vi "feedback.vi"(3 "Dataflow In":errorcluster) -> (1 "Dataflow Out":errorcluster)   [LabVIEW 2019]
uses:
  lib/libSimulationControl/libSimulationControl.lvlib
panel:
  # "*******************************************************************\nBiogas Plant Control\n\nAuthor: Paul Zügel\nGCSC-Frankfurt am Main 2020\n\n*******************************************************************"
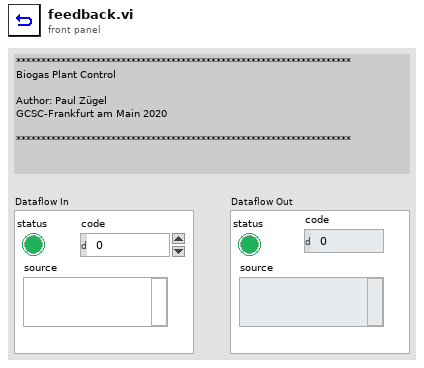
[diagram p1: front panel]
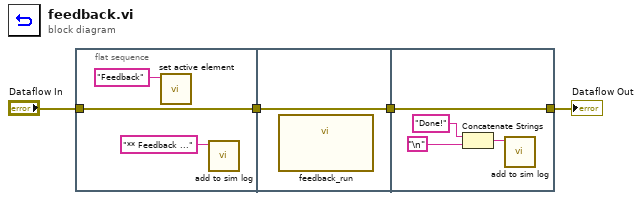
[diagram p0: block diagram]
diagram:
  n1 = flat-sequence {
    tunnel: "Dataflow In" -> [w5]
    tunnel: [w5] -> w4
    tunnel: [w8] -> w3
    tunnel: w4 -> [w8]
    tunnel: [w12] -> w1
    tunnel: w3 -> [w12]
    frame #0 {
      n2 = call "set active element.vi"("elem"="Feedback") -> ()  [unwired: 10 in, 1 out]
      n3 = call "add to sim log.vi"("log"="** Feedback ..." ("string")) -> ()  [unwired: 10 in, 1 out]
    }
    frame #1 {
      n4 = call "feedback_run.vi"() -> ()  [unwired: 12 in]
    }
    frame #2 {
      n5 = Concatenate Strings("Done!" ("string"), "\n") -> (w9:string)
      n6 = call "add to sim log.vi"("log"=w9) -> ()  [unwired: 10 in, 1 out]
    }
  }
  "Dataflow Out" <- w1
